vi "Práctica11_GPIB.vi"() -> ()   [LabVIEW 2021]
uses:
  <vilib>/Instr/_visa.llb/GPIB Status Boolean Array.ctl
panel:
  out "error out 2":errorcluster
  out "byte count 2":i32
  out "GPIB error":i16
  in  "byte count":i32
  in  "error in":errorcluster
  in  "system controller (T)":bool
  in  "data":string
  in  "address string":string
  out "ibsta 2":T1
  out "ibsta":T1
  out "error out":errorcluster
  # "Anahí Montserrat Vázquez Padilla\nComunicación por GPIB\n30/04/2024"
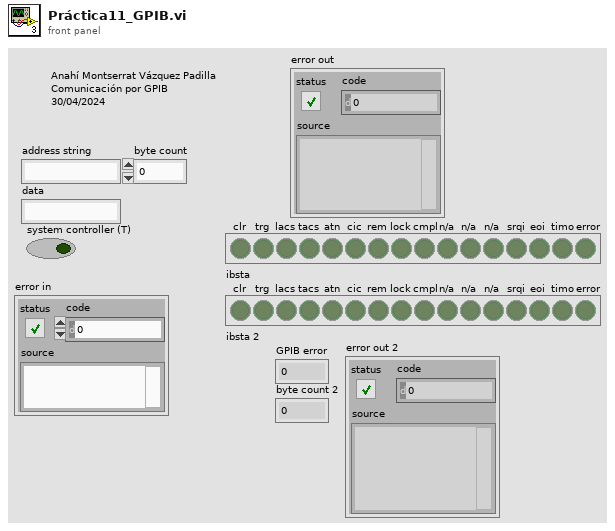
[diagram p1: front panel]
types:
  T1 = typedef "GPIB Status Boolean Array.ctl" = bool[]
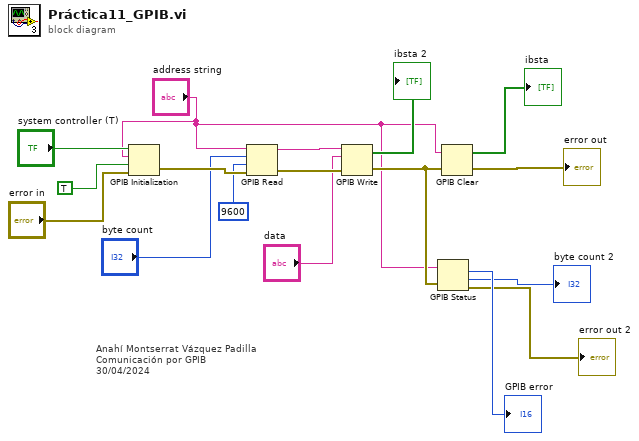
[diagram p0: block diagram]
diagram:
  # "Anahí Montserrat Vázquez Padilla\nComunicación por GPIB\n30/04/2024"
  n1 = GPIB Initialization(4:"error in", 5:TRUE, 6:"address string", 7:"system controller (T)") -> (0:w13:errorcluster)  [unwired: 3 in]
  n2 = GPIB Read(0:"address string", 1:"byte count", 2:9600, 3:w13) -> (5:w14:string, 7:w12:errorcluster)  [unwired: 1 in, 1 out]
  n3 = GPIB Write(0:w14, 1:"data", 3:w12) -> (5:→"ibsta 2":bool[], 6:w10:errorcluster)  [unwired: 2 in]
  n4 = GPIB Status(0:"address string", 1:w10) -> (3:→"GPIB error":i16, 4:→"byte count 2":i32, 5:→"error out 2":errorcluster)  [unwired: 1 out]
  n5 = GPIB Clear(2:w10, 3:"address string") -> (0:→"error out":errorcluster, 1:→"ibsta":bool[])
